vi "Error - Fire Error.vi"(8 "error in (no error)":errorcluster, 10 "Error Type":T1, 11 "View Model":T2) -> (0 "error out":errorcluster, 3 "View Model":T2)   [LabVIEW 2017]
doc: "Generates error with parameters"
uses:
  View Model/Controls/View Model.ctl
  Configuration Database/Controls/Config Model.ctl
  Configuration Database/Controls/Congif Data.ctl
  Configuration Database/Controls/Config Commands.ctl
  View Model/Controls/Shared Model.ctl
  Controls/Error Model.ctl
  Controls/Error Data.ctl
  Controls/Error Type.ctl
  Car Wash Controller/Controls/Car Wash Model.ctl
  Views/Entry Console View/Controls/Entry Console Data.ctl
panel:
  # "[Covers: EH1]"
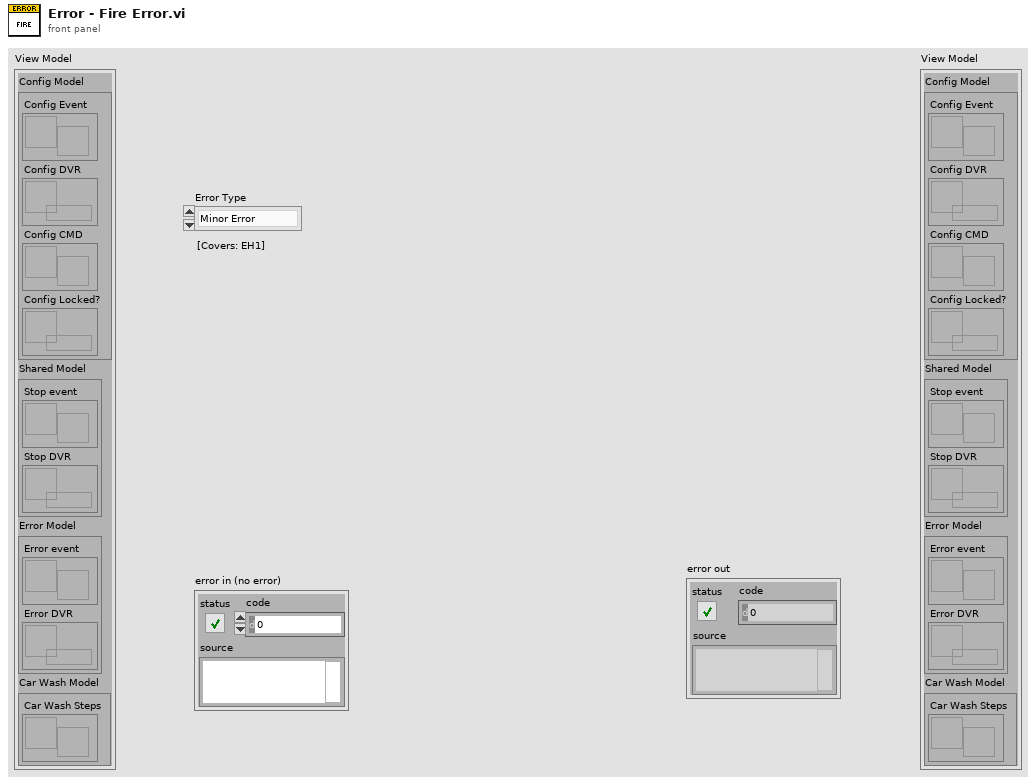
[diagram p1: front panel]
types:
  T1 = typedef "Error Type.ctl" = enum16{"Minor Error", "Wash Cycle Error", "System Error", "Other Error"}
  T2 = typedef "View Model.ctl" = cluster{"Config Model":T3, "Shared Model":T4, "Error Model":T5, "Car Wash Model":T6}
  T3 = typedef "Config Model.ctl" = cluster{"Config Event":refnum<user-event>, "Config DVR":refnum<data-value>, "Config CMD":refnum<user-event>, "Config Locked?":refnum<data-value>}
  T4 = typedef "Shared Model.ctl" = cluster{"Stop event":refnum<user-event>, "Stop DVR":refnum<data-value>}
  T5 = typedef "Error Model.ctl" = cluster{"Error event":refnum<user-event>, "Error DVR":refnum<data-value>}
  T6 = typedef "Car Wash Model.ctl" = cluster{"Car Wash Steps":refnum<user-event>}
  T7 = typedef "Error Data.ctl" = cluster{"Error Type":T1, "Error cluster":errorcluster, "Other Data":variant}
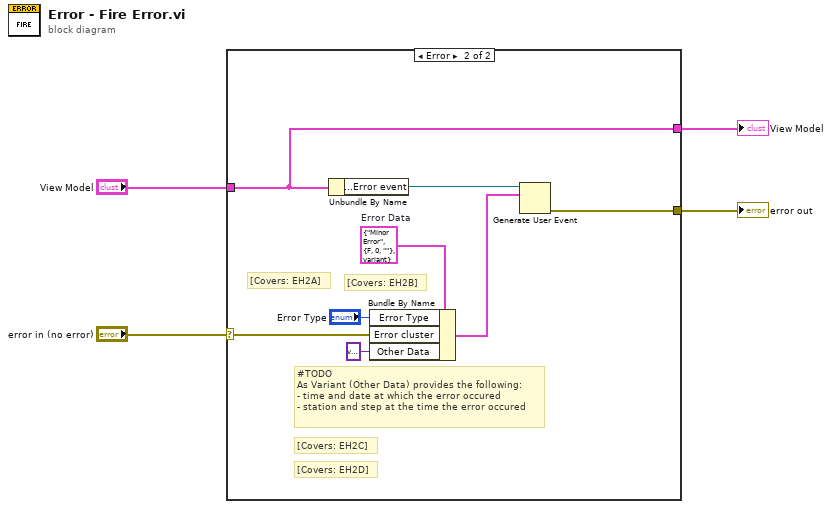
[diagram p0: block diagram]
diagram:
  n1 = case shown="Error" "error in (no error)" {
    selector: "error in (no error)" -> [w5 w10]
    tunnel: "View Model" -> [w6 w13]
    tunnel: [w6 w13] -> w2
    tunnel: [w5 w8] -> w1
    frame No Error {
    }
    frame Error {
      w12 = T7 {"Error Type"=enum."Minor Error", "Error cluster"={"status"=FALSE, "code"=0, "source"=""}, "Other Data"=variant}  # Error Data
      # "[Covers: EH2A]"
      # "[Covers: EH2B]"
      # "[Covers: EH2D]"
      # "[Covers: EH2C]"
      # "#TODO\nAs Variant (Other Data) provides the following:\n- time and date at which the error occured\n- station and step at the time the error occured"
      n2 = Unbundle By Name(w13) -> ("Error Model.Error event"=w14:refnum<user-event>)
      n3 = Bundle By Name(cluster=w12, "Error Type"="Error Type", "Error cluster"=w10, "Other Data"=variant) -> (w11:T7)
      n4 = Generate User Event(user event=w14, event data cluster=w11) -> (error out=w8:errorcluster)  [unwired: 2 in, 1 out]
    }
  }
  "View Model" <- w2
  "error out" <- w1
